vi "example fpga code.vi"() -> ()   [LabVIEW 2014]
uses:
  Shared/UEGO fpga outputs.ctl
  Shared/UEGO fpga inputs.ctl
  <vilib>/rvi/Emulation/niFpgaGetClockAttributes.vi
  <vilib>/rvi/Emulation/niFpgaSctlEmulationGetInTimedLoop.vi
  <vilib>/rvi/Emulation/niFpgaEmulationReportErrorSimple.vi
  <vilib>/rvi/eio/common/nirviEmuTemplateMethod_errors.vi
  <vilib>/rvi/Emulation/niFpgaCriticalErrorInLSC.vi
  <vilib>/eio/EIONode/EIONode.xnode
  <vilib>/NI Veristand/FPGA/NI_VS FPGA Support.lvlib
  Shared/UEGO Sim Shared.lvlib
panel:
  in  "UEGO.4.out":T1={"Sensor Model"=enum."Narrow Band", "lambda"=1.0, "cal"=FALSE, "negate"=FALSE, "PWM threshold"=1500, "PWM timeout"=40000}
  in  "UEGO.3.out":T1={"Sensor Model"=enum."Narrow Band", "lambda"=1.0, "cal"=FALSE, "negate"=FALSE, "PWM threshold"=1500, "PWM timeout"=40000}
  out "UEGO.4.in":T3
  out "UEGO.3.in":T3
  out "UEGO.2.in":T3
  in  "UEGO.2.out":T1={"Sensor Model"=enum."Narrow Band", "lambda"=1.0, "cal"=FALSE, "negate"=FALSE, "PWM threshold"=1500, "PWM timeout"=40000}
  out "UEGO.1.in":T3
  in  "UEGO.1.out":T1={"Sensor Model"=enum."Narrow Band", "lambda"=1.0, "cal"=FALSE, "negate"=FALSE, "PWM threshold"=1500, "PWM timeout"=40000}
  out "Iteration time (ticks)":u32
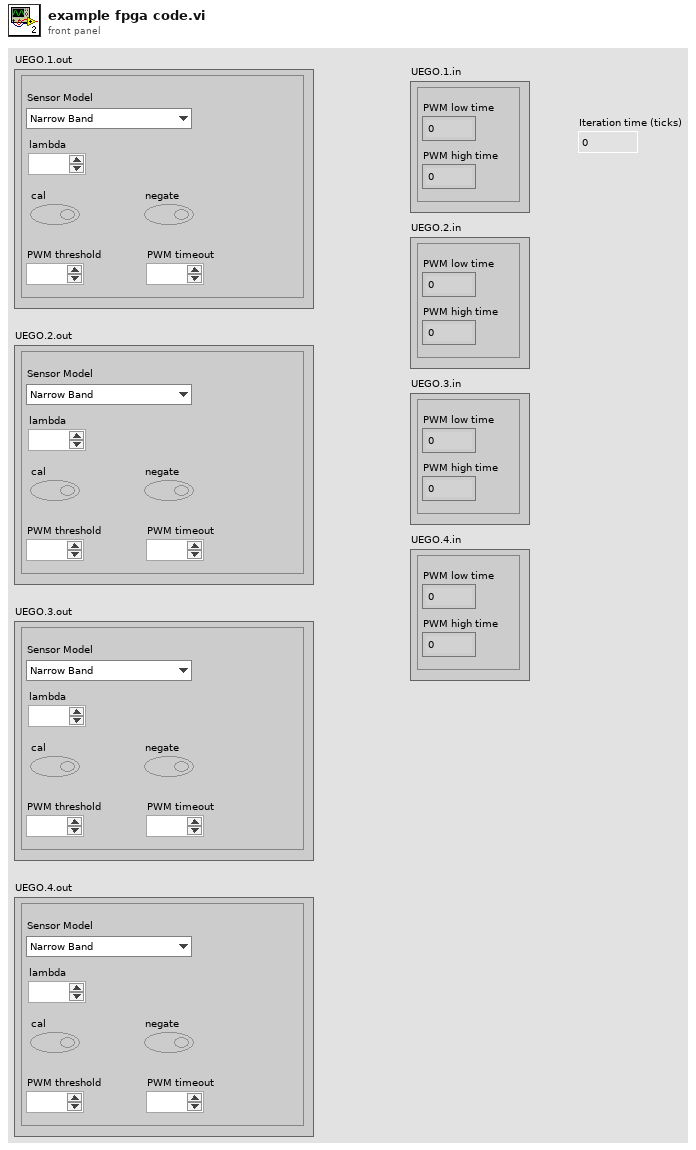
[diagram p1: front panel]
types:
  T1 = typedef "UEGO Sim Shared.lvlib/UEGO fpga outputs.ctl" = cluster{"Sensor Model":T2, "lambda":fxp<+,12,3>, "cal":bool, "negate":bool, "PWM threshold":i16, "PWM timeout":u32}
  T2 = typedef "UEGO Sim Shared.lvlib/sensor models" = enum16{"Narrow Band", "Bosch 4.2", "Bosch 4.9"}
  T3 = typedef "UEGO Sim Shared.lvlib/UEGO fpga inputs.ctl" = cluster{"PWM low time":u32, "PWM high time":u32}
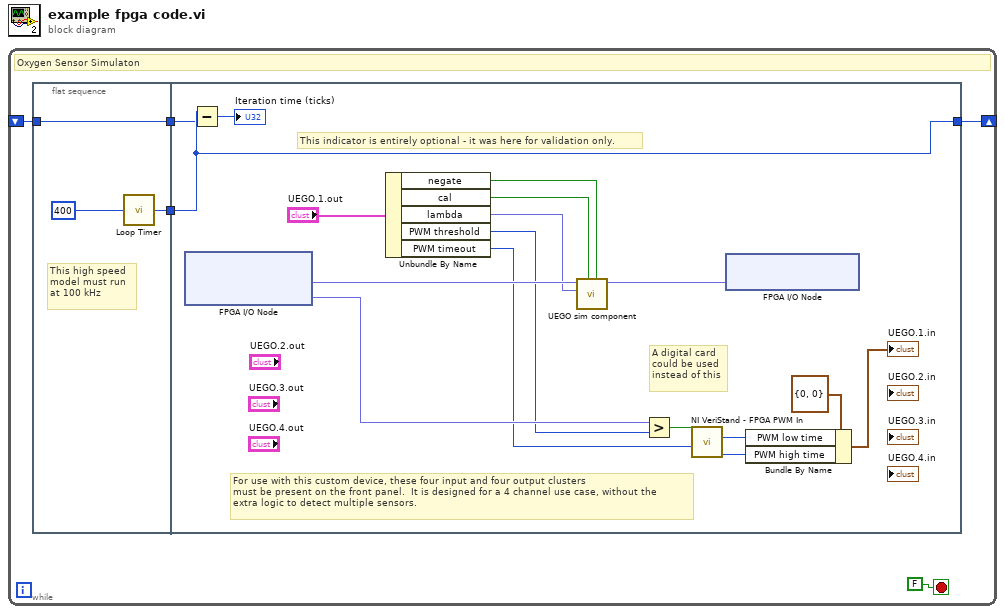
[diagram p0: block diagram]
diagram:
  n1 = while {
    shift-right: [w3] -> _
    shift-left: _ -> [w1]
    stop <- FALSE stop-if-true
    # "Oxygen Sensor Simulaton"
    n2 = flat-sequence {
      tunnel: [w7] -> w4
      tunnel: [w6] -> w2
      tunnel: w1 -> [w6]
      tunnel: w4 -> [w25]
      tunnel: [w25] -> w3
      tunnel: w2 -> [w24]
      frame #0 {
        # "This high speed\nmodel must run\nat 100 kHz"
        n3 = call "Loop Timer"("Count(Ticks)"=u32 400 ("Period (ticks)")) -> ("Tick Count(Ticks)"=w7:u32)
      }
      frame #1 {
        # "For use with this custom device, these four input and four output clusters\nmust be present on the front panel.  It is designed for a 4 channel use case, without the \nextra logic to detect multiple sensors."
        # "This indicator is entirely optional - it was here for validation only."
        # "A digital card\ncould be used\ninstead of this"
        n4 = xnode "FPGA I/O Node"() -> ("Connector1/AI0"=w19:fxp<+/-,27,5>, "Connector1/AI1"=w21:fxp<+/-,27,5>)  [unwired: 2 in, 2 out]
        n5 = Subtract(x=w25, y=w24) -> (x-y=→"Iteration time (ticks)":u32)
        n6 = Unbundle By Name("UEGO.1.out") -> ("negate"=w15:bool, "cal"=w16:bool, "lambda"=w17:fxp<+,12,3>, "PWM threshold"=w11:i16, "PWM timeout"=w14:u32)
        n7 = call "UEGO sim component.vi"("UEGO.1.negate"=w15, "UEGO.1.cal"=w16, "UEGO.1.lambda"=w17, "AI in"=w19) -> ("AO out"=w20:fxp<+/-,37,21>)  [unwired: 7 in]
        n8 = Greater?(x=w21, y=w11) -> (0:w22:bool)
        n9 = call <vilib>:"NI VeriStand - FPGA PWM In.vi"("Time Out"=w14, "Value"=w22) -> ("High time"=w12:u32, "Low Time"=w13:u32)  [unwired: 8 out]
        n10 = xnode "FPGA I/O Node"("Connector1/AO0"=w20) -> ()  [unwired: 1 in, 1 out]
        n11 = Bundle By Name(cluster=T3 {"PWM low time"=0, "PWM high time"=0} ("UEGO.1.in"), "PWM low time"=w13, "PWM high time"=w12) -> (→"UEGO.1.in":T3)
      }
    }
  }
